vi "Teleop.vi"(10 "Match Info":T1={"Autonomous Elapsed Seconds"=0.0, "TeleOp Elapsed Seconds"=0.0, "Disabled Elapsed Seconds"=0.0, "Visited Autonomous"=FALSE, "Visited TeleOp"=FALSE, "Visited Disabled"=FALSE, "Autonomous Settings"={"Autonomous Style"=enum."Independent", "VI Refnum"=refnum}}, 11 "Call Context":T2) -> ()   [LabVIEW 2012]
doc: "This VI is called for each TeleOp packet received from the DS where the robot is not disabled. It is often used to read from the joysticks and update I/O or to update setpoints for timed control loops. It should complete and return within 20 milliseconds or it may miss DS packets."
uses:
  <vilib>/Rock Robotics/WPI/DriverStation/WPI_DriverStationDerivedRobotMode.ctl
  <vilib>/Rock Robotics/WPI/DriverStation/WPI_DriverStationMatch Info.ctl
  <vilib>/Rock Robotics/WPI/Relay/WPI_RelayValue.ctl
  Robot Global Data.vi
  <vilib>/Rock Robotics/WPI/Joystick/WPI_JoystickGetSetRefNum.vi
panel:
  in  "Ext Const":dbl=0.5
  in  "Dep Const":dbl=1.0
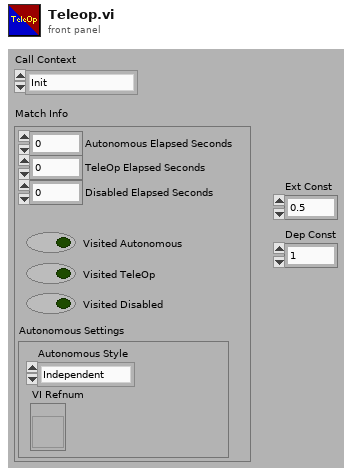
[diagram p1: front panel]
types:
  T1 = typedef "WPI_DriverStationMatch Info.ctl" = cluster{"Autonomous Elapsed Seconds":dbl, "TeleOp Elapsed Seconds":dbl, "Disabled Elapsed Seconds":dbl, "Visited Autonomous":bool, "Visited TeleOp":bool, "Visited Disabled":bool, "Autonomous Settings":cluster{"Autonomous Style":enum16{"Iterative", "Independent"}, "VI Refnum":refnum<vi>}}
  T2 = typedef "WPI_DriverStationDerivedRobotMode.ctl" = enum16{"Init", "Execute", "Stop"}
  T3 = typedef "WPI_RelayValue.ctl" = enum16{"Off", "On", "Forward", "Reverse"}
  T4 = cluster{"Driver Station Digital Input (1-8)[0]":bool, "Driver Station Digital Input (1-8)[1]":bool, "Driver Station Digital Input (1-8)[2]":bool, "Driver Station Digital Input (1-8)[3]":bool, "Driver Station Digital Input (1-8)[4]":bool, "Driver Station Digital Input (1-8)[5]":bool, "Driver Station Digital Input (1-8)[6]":bool, "Driver Station Digital Input (1-8)[7]":bool, "Driver Station Digital Input (1-8)[8]":bool}
  T5 = cluster{"Right Servo High":dbl, "Right Servo Mid":dbl, "Right Servo Low":dbl, "Left Servo High":dbl, "Left Servo Mid":dbl, "Left Servo Low":dbl}
  T6 = typedef "WPI_JoystickDevRef.ctl" = cluster{"Device":T7}
  T7 = typedef "WPI_JoystickDeviceEnum.ctl" = enum16{"USB 1", "USB 2", "USB 3", "USB 4", "Kinect 1", "Kinect 2"}
  T8 = cluster{"axis 1 (x)":dbl, "axis 2 (y)":dbl, "axis 3 (throttle)":dbl, "axis 4":dbl, "axis 5":dbl, "axis 6":dbl}
  T9 = typedef "WPI_ServoDeviceRef.ctl" = cluster{"DeviceStatus":errorcluster, "Digital Module":T10, "PWM Channel":T11, "DeadBand":T12}
  T10 = typedef "FPGA_TypedefDigitalModule.ctl" = enum16{"Digital Module 1", "Digital Module 2"}
  T11 = typedef "FPGA_DIOPWMChannel.ctl" = enum8{"PWM 1", "PWM 2", "PWM 3", "PWM 4", "PWM 5", "PWM 6", "PWM 7", "PWM 8", "PWM 9", "PWM 10", "Invalid"}
  T12 = typedef "WPI_PWMDeadband.ctl" = cluster{"Name":string, "maxPositivePwm":i32, "minPositivePwm":i32, "centerPwm":i32, "maxNegativePwm":i32, "minNegativePwm":i32, "angularRange":u16}
  T13 = typedef "WPI_MotorControlDeviceRef.ctl" = cluster{"DeviceStatus":errorcluster, "Type":enum16{"PWM", "CAN"}, "PWM":cluster{"Digital Module":T10, "PWM Channel":T11, "DeadBand":T12}, "CAN":cluster{"Device Number":u8, "Control Mode":T14, "Semaphore":T15, "Max Vout":dbl}, "Invert":bool, "TransformRef":T16, "InvTransformRef":T16}
  T14 = typedef "WPI_CANJaguar_ControlMode.ctl" = enum8{"Percent VBus", "Current", "Speed", "Position", "Voltage"}
  T15 = typedef "Semaphore RefNum" = refnum<k1>
  T16 = typedef "WPI_PWMTransform_ConPane.ctl" = refnum<vi>
  T17 = typedef "WPI_JoystickButtonState.ctl" = cluster{"Button 1":bool, "Button 2":bool, "Button 3":bool, "Button 4":bool, "Button 5":bool, "Button 6":bool, "Button 7":bool, "Button 8":bool, "Button 9":bool, "Button 10":bool, "Button 11":bool, "Button 12":bool}
  T18 = cluster{"FlipperLeftUp":dbl, "FlipperLeftDown":dbl, "FlipperRightUp":dbl, "FlipperRightDown":dbl, "KickerLeftBack":dbl, "KickerLeftForward":dbl, "KickerRightBack":dbl, "KickerRightForward":dbl}
  T19 = typedef "WPI_RelayDevRef.ctl" = cluster{"DevStatus":errorcluster, "Relay Channel":T20, "Digital Module":T10, "Relay Direction":T21}
  T20 = typedef "FPGA_DIORelayChannel.ctl" = enum8{"Relay 1", "Relay 2", "Relay 3", "Relay 4", "Relay 5", "Relay 6", "Relay 7", "Relay 8", "Invalid"}
  T21 = typedef "WPI_RelayDirection.ctl" = enum16{"Both directions", "Forward only", "Reverse only"}
  T22 = typedef "WPI_DigitalInputDevRef.ctl" = cluster{"DevStatus":errorcluster, "DIO Channel":T23, "Digital Module":T10}
  T23 = typedef "FPGA_DIOChannel.ctl" = enum8{"DIO 1", "DIO 2", "DIO 3", "DIO 4", "DIO 5", "DIO 6", "DIO 7", "DIO 8", "DIO 9", "DIO 10", "DIO 11", "DIO 12", "DIO 13", "DIO 14", "Invalid"}
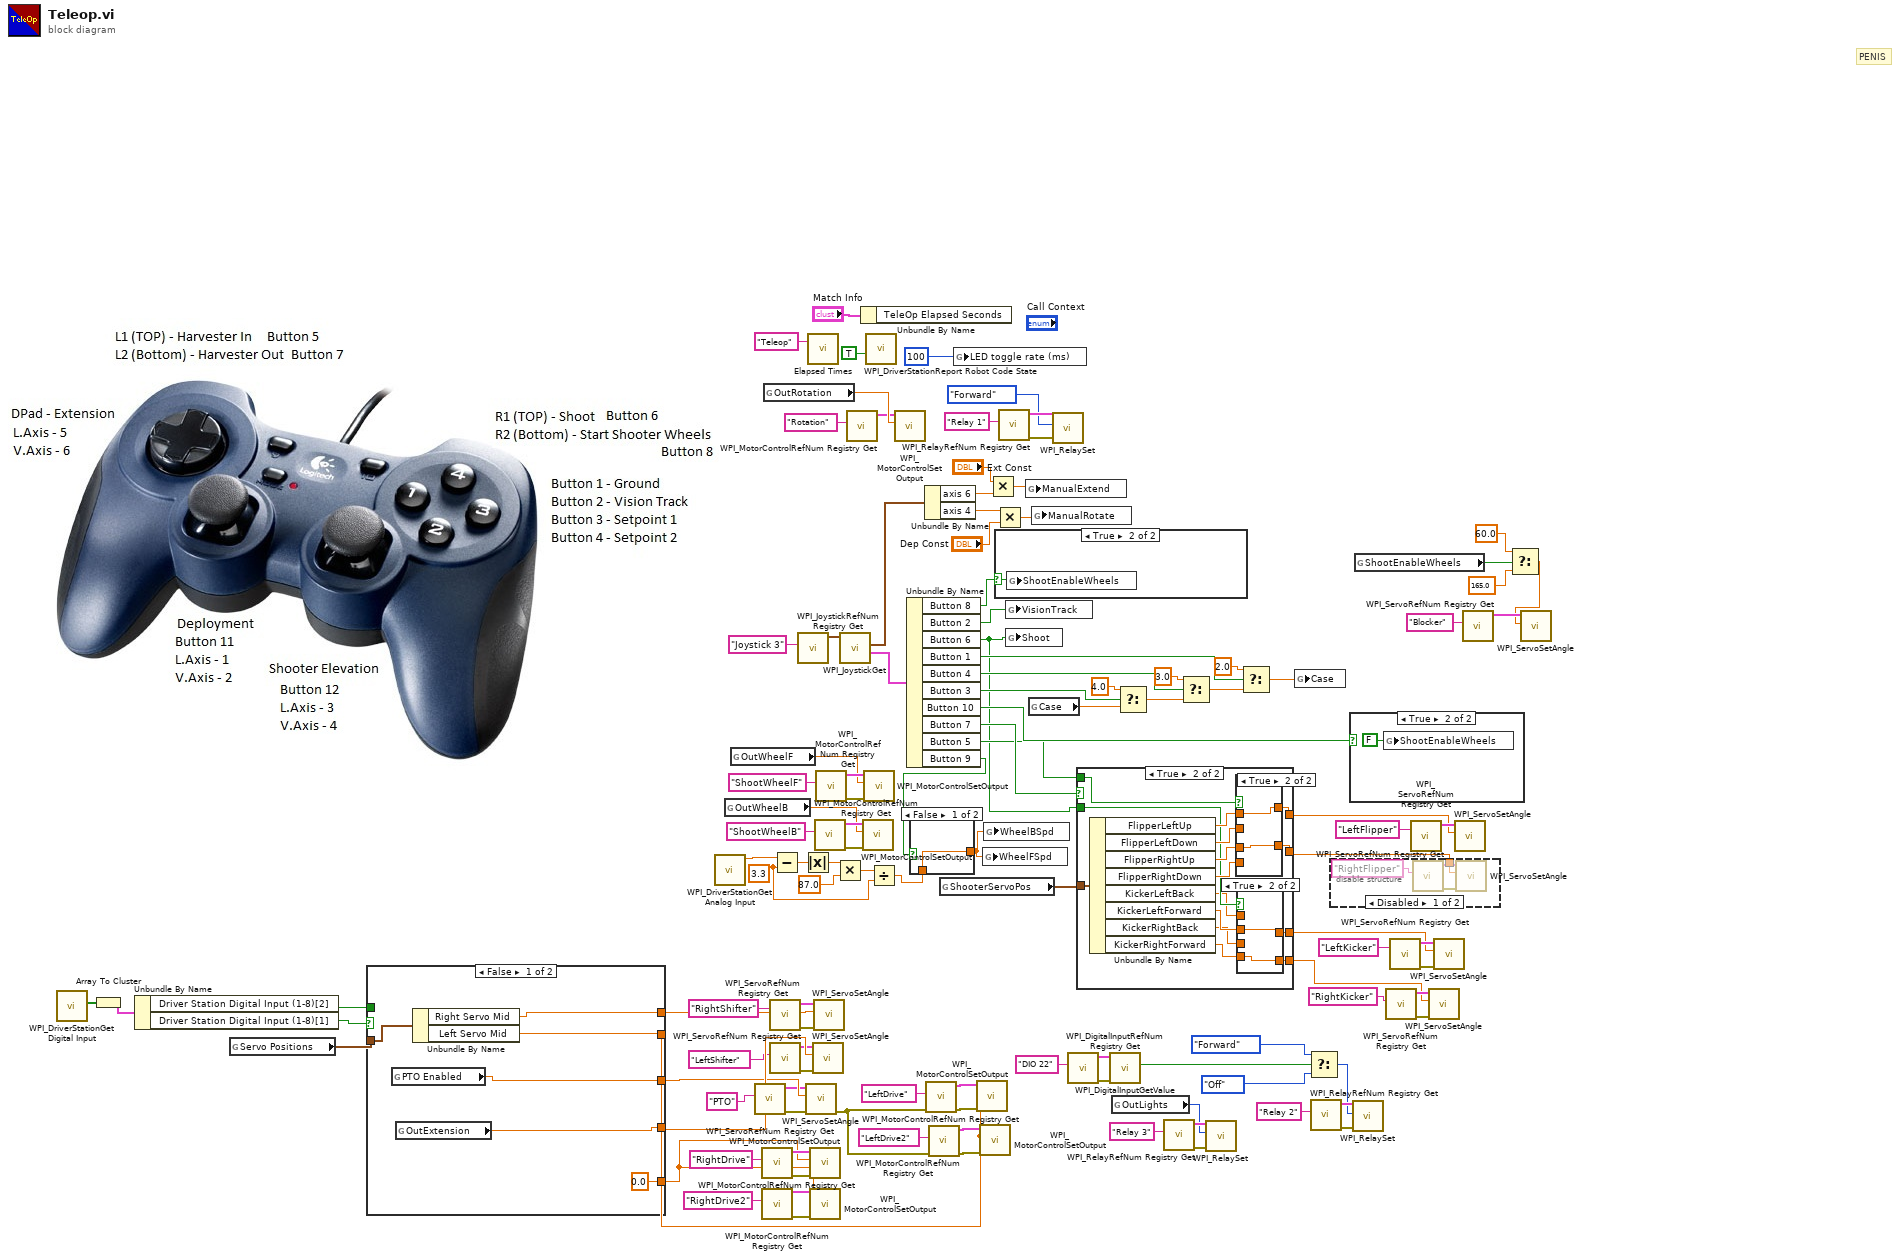
[diagram p0: block diagram]
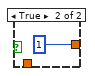
[diagram p2: hidden frame]
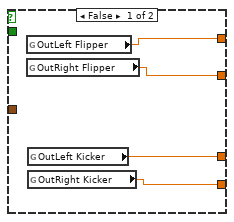
[diagram p4: hidden frame]
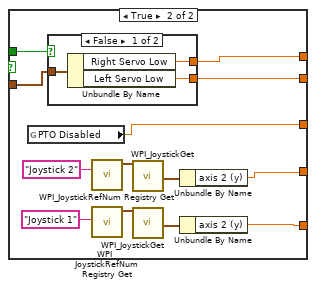
[diagram p7: hidden frame]
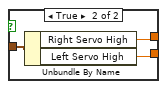
[diagram p8: hidden frame]
diagram:
  w2 = 3.3 ("y")
  # "PENIS"
  n1 = call <vilib>:"WPI_DriverStationGet Digital Input.vi"() -> ("Driver Station Digital Input (1-8)"=w87:bool[])  [unwired: 11 in]
  n2 = Array To Cluster(array=w87) -> (cluster=w86:T4)
  n3 = Unbundle By Name(w86) -> ("Driver Station Digital Input (1-8)[2]"=w85:bool, "Driver Station Digital Input (1-8)[1]"=w25:bool)
  n4 = global read "Robot Global Data.vi" "Servo Positions"() -> (w84:T5)
  n5 = case shown="False" w25 {
    tunnel: w85 -> [_ w138]
    tunnel: w84 -> [w125 w137]
    tunnel: [w124 w136] -> w83
    tunnel: [w123 w135] -> w82
    tunnel: [w122 w134] -> w75
    tunnel: [w120 w127] -> w74
    tunnel: [0.0 w126] -> w73
    frame False {
      n6 = global read "Robot Global Data.vi" "PTO Enabled"() -> (w122:dbl)
      n7 = global read "Robot Global Data.vi" "OutExtension"() -> (w120:dbl)
      n8 = Unbundle By Name(w125) -> ("Right Servo Mid"=w124:dbl, "Left Servo Mid"=w123:dbl)
    }
    frame True {
      n9 = global read "Robot Global Data.vi" "PTO Disabled"() -> (w134:dbl)
      n10 = case shown="False" w138 {
        tunnel: w137 -> [w141 w144]
        tunnel: [w140 w143] -> w136
        tunnel: [w139 w142] -> w135
        frame False {
          n11 = Unbundle By Name(w141) -> ("Right Servo Low"=w140:dbl, "Left Servo Low"=w139:dbl)
        }
        frame True {
          n12 = Unbundle By Name(w144) -> ("Right Servo High"=w143:dbl, "Left Servo High"=w142:dbl)
        }
      }
      n13 = call <vilib>:"WPI_JoystickRefNum Registry Get.vi"("refnum name"="Joystick 2") -> ("JoystickDevRef"=w128:T6)  [unwired: 1 in, 9 out]
      n14 = call <vilib>:"WPI_JoystickRefNum Registry Get.vi"("refnum name"="Joystick 1") -> ("JoystickDevRef"=w132:T6)  [unwired: 1 in, 9 out]
      n15 = call <vilib>:"WPI_JoystickGet.vi"("JoystickDevRef"=w128) -> ("Axes"=w130:T8)  [unwired: 1 in, 5 out]
      n16 = call <vilib>:"WPI_JoystickGet.vi"("JoystickDevRef"=w132) -> ("Axes"=w133:T8)  [unwired: 1 in, 5 out]
      n17 = Unbundle By Name(w130) -> ("axis 2 (y)"=w127:dbl)
      n18 = Unbundle By Name(w133) -> ("axis 2 (y)"=w126:dbl)
    }
  }
  n19 = call <vilib>:"WPI_DriverStationGet Analog Input.vi"() -> ("Analog 1 (V)"=w7:dbl)  [unwired: 8 in, 3 out]
  n20 = global read "Robot Global Data.vi" "OutWheelB"() -> (w45:dbl)
  n21 = global read "Robot Global Data.vi" "OutWheelF"() -> (w46:dbl)
  n22 = call <vilib>:"WPI_ServoRefNum Registry Get.vi"("refnum name"="PTO") -> ("error out"=w68:errorcluster, "ServoDeviceRef"=w69:T9)  [unwired: 9 in]
  n23 = call <vilib>:"WPI_MotorControlRefNum Registry Get.vi"("refnum name"="RightDrive") -> ("error out"=w97:errorcluster, "MotorControlDevRef"=w99:T13)  [unwired: 9 in]
  n24 = call <vilib>:"WPI_MotorControlRefNum Registry Get.vi"("refnum name"="RightDrive2") -> ("error out"=w90:errorcluster, "MotorControlDevRef"=w88:T13)  [unwired: 9 in]
  n25 = global read "Robot Global Data.vi" "OutRotation"() -> (w72:dbl)
  n26 = call <vilib>:"WPI_ServoRefNum Registry Get.vi"("refnum name"="RightShifter") -> ("error out"=w78:errorcluster, "ServoDeviceRef"=w79:T9)  [unwired: 9 in]
  n27 = call <vilib>:"WPI_ServoRefNum Registry Get.vi"("refnum name"="LeftShifter") -> ("error out"=w80:errorcluster, "ServoDeviceRef"=w81:T9)  [unwired: 9 in]
  n28 = Subtract(x=w7, y=w2) -> (x-y=w6:dbl)
  n29 = call <vilib>:"WPI_JoystickRefNum Registry Get.vi"("refnum name"="Joystick 3") -> ("JoystickDevRef"=w116:T6)  [unwired: 9 in, 1 out]
  n30 = Absolute Value(x=w6) -> (abs(x)=w5:dbl)
  n31 = call <vilib>:"WPI_ServoSetAngle.vi"("error in (no error)"=w68, "Angle"=w75, "ServoDeviceRef"=w69) -> ("error out"=w64:errorcluster)  [unwired: 7 in, 1 out]
  n32 = call "Elapsed Times.vi"("Call Name"="Teleop") -> ()  [unwired: 2 in, 1 out]
  n33 = call <vilib>:"WPI_MotorControlSetOutput.vi"("error in (no error)"=w97, "Output"=w73, "MotorControlDevRef"=w99) -> ()  [unwired: 6 in, 3 out]
  n34 = call <vilib>:"WPI_MotorControlSetOutput.vi"("error in (no error)"=w90, "Output"=w73, "MotorControlDevRef"=w88) -> ()  [unwired: 6 in, 3 out]
  n35 = call <vilib>:"WPI_ServoSetAngle.vi"("error in (no error)"=w80, "Angle"=w82, "ServoDeviceRef"=w81) -> ()  [unwired: 7 in, 2 out]
  n36 = call <vilib>:"WPI_ServoSetAngle.vi"("error in (no error)"=w78, "Angle"=w83, "ServoDeviceRef"=w79) -> ()  [unwired: 7 in, 2 out]
  n37 = call <vilib>:"WPI_MotorControlRefNum Registry Get.vi"("refnum name"="ShootWheelB") -> ("error out"=w48:errorcluster, "MotorControlDevRef"=w49:T13)  [unwired: 9 in]
  n38 = call <vilib>:"WPI_MotorControlRefNum Registry Get.vi"("refnum name"="ShootWheelF") -> ("error out"=w50:errorcluster, "MotorControlDevRef"=w47:T13)  [unwired: 9 in]
  n39 = Multiply(x=w5, y=87.0) -> (x*y=w3:dbl)
  n40 = call <vilib>:"WPI_JoystickGet.vi"("JoystickDevRef"=w116) -> ("Buttons"=w114:T17, "Axes"=w113:T8)  [unwired: 4 in, 1 out]
  n41 = call <vilib>:"WPI_MotorControlRefNum Registry Get.vi"("refnum name"="Rotation") -> ("MotorControlDevRef"=w70:T13)  [unwired: 9 in, 1 out]
  n42 = Unbundle By Name("Match Info") -> ()  [unwired: 1 out]
  n43 = call <vilib>:"WPI_MotorControlSetOutput.vi"("error in (no error)"=w48, "Output"=w45, "MotorControlDevRef"=w49) -> ()  [unwired: 6 in, 3 out]
  n44 = call <vilib>:"WPI_MotorControlSetOutput.vi"("error in (no error)"=w50, "Output"=w46, "MotorControlDevRef"=w47) -> ()  [unwired: 6 in, 3 out]
  n45 = call <vilib>:"WPI_DriverStationReport Robot Code State.vi"("TeleOp"=TRUE ("Autonomous")) -> ()  [unwired: 10 in, 1 out]
  n46 = Divide(x=w3, y=w2) -> (x/y=w1:dbl)
  n47 = call <vilib>:"WPI_MotorControlSetOutput.vi"("Output"=w72, "MotorControlDevRef"=w70) -> ()  [unwired: 7 in, 3 out]
  n48 = Unbundle By Name(w114) -> ("Button 8"=w101:bool, "Button 2"=w112:bool, "Button 6"=w29:bool, "Button 1"=w111:bool, "Button 4"=w109:bool, "Button 3"=w108:bool, "Button 10"=w44:bool, "Button 7"=w43:bool, "Button 5"=w42:bool, "Button 9"=w26:bool)
  n49 = case shown="False" w26 {
    tunnel: [w145 1] -> w27
    tunnel: w1 -> [w145 _]
    frame False {
    }
    frame True {
    }
  }
  n50 = Unbundle By Name(w113) -> ("axis 6"=w55:dbl, "axis 4"=w65:dbl)
  n51 = call <vilib>:"WPI_MotorControlRefNum Registry Get.vi"("error in (no error)"=w64, "refnum name"="LeftDrive") -> ("error out"=w92:errorcluster, "MotorControlDevRef"=w95:T13)  [unwired: 8 in]
  n52 = call <vilib>:"WPI_MotorControlRefNum Registry Get.vi"("error in (no error)"=w64, "refnum name"="LeftDrive2") -> ("error out"=w91:errorcluster, "MotorControlDevRef"=w93:T13)  [unwired: 8 in]
  n53 = global read "Robot Global Data.vi" "ShooterServoPos"() -> (w30:T18)
  n54 = global write "Robot Global Data.vi" "LED toggle rate (ms)"(u32 100 ("LED ms toggle rate")) -> ()
  n55 = call <vilib>:"WPI_MotorControlSetOutput.vi"("error in (no error)"=w92, "Output"=w74, "MotorControlDevRef"=w95) -> ()  [unwired: 6 in, 3 out]
  n56 = call <vilib>:"WPI_MotorControlSetOutput.vi"("error in (no error)"=w91, "Output"=w74, "MotorControlDevRef"=w93) -> ()  [unwired: 6 in, 3 out]
  n57 = global write "Robot Global Data.vi" "WheelFSpd"(w27) -> ()
  n58 = global write "Robot Global Data.vi" "WheelBSpd"(w27) -> ()
  n59 = Multiply(x="Ext Const", y=w55) -> (x*y=w53:dbl)
  n60 = Multiply(x=w65, y="Dep Const") -> (x*y=w63:dbl)
  n61 = case shown="True" w101 {
    selector: w101 -> [_ w147]
    frame False {
    }
    frame True {
      n62 = global write "Robot Global Data.vi" "ShootEnableWheels"(w147) -> ()
    }
  }
  n63 = call <vilib>:"WPI_RelayRefNum Registry Get.vi"("refnum name"="Relay 1") -> ("error out"=w60:errorcluster, "RelayDevRef"=w62:T19)  [unwired: 9 in]
  n64 = global write "Robot Global Data.vi" "VisionTrack"(w112) -> ()
  n65 = global write "Robot Global Data.vi" "Shoot"(w29) -> ()
  n66 = global write "Robot Global Data.vi" "ManualExtend"(w53) -> ()
  n67 = global read "Robot Global Data.vi" "Case"() -> (w103:dbl)
  n68 = global write "Robot Global Data.vi" "ManualRotate"(w63) -> ()
  n69 = call <vilib>:"WPI_RelaySet.vi"("error in (no error)"=w60, "RelayValue"=WPI_RelayValue."Forward", "RelayDevRef"=w62) -> ()  [unwired: 7 in, 2 out]
  n70 = call <vilib>:"WPI_DigitalInputRefNum Registry Get.vi"("refnum name"="DIO 22") -> ("error out"=w19:errorcluster, "DigitalInputDevRef"=w15:T22)  [unwired: 9 in]
  n71 = case shown="True" w43 {
    tunnel: w42 -> [_ w152]
    tunnel: [w151 w165] -> w33
    tunnel: [w150 w163] -> w32
    tunnel: [w149 w154] -> w31
    tunnel: [w148 w153] -> w28
    tunnel: w30 -> [_ w166]
    tunnel: w29 -> [_ w159]
    frame False {
      n72 = global read "Robot Global Data.vi" "OutLeft Flipper"() -> (w151:dbl)
      n73 = global read "Robot Global Data.vi" "OutRight Flipper"() -> (w150:dbl)
      n74 = global read "Robot Global Data.vi" "OutLeft Kicker"() -> (w149:dbl)
      n75 = global read "Robot Global Data.vi" "OutRight Kicker"() -> (w148:dbl)
    }
    frame True {
      n76 = Unbundle By Name(w166) -> ("FlipperLeftUp"=w164:dbl, "FlipperLeftDown"=w161:dbl, "FlipperRightUp"=w162:dbl, "FlipperRightDown"=w160:dbl, "KickerLeftBack"=w158:dbl, "KickerLeftForward"=w157:dbl, "KickerRightBack"=w156:dbl, "KickerRightForward"=w155:dbl)
      n77 = case shown="True" w152 {
        tunnel: [w172 w174] -> w165
        tunnel: w164 -> [_ w174]
        tunnel: [w171 w173] -> w163
        tunnel: w162 -> [_ w173]
        tunnel: w161 -> [w172 _]
        tunnel: w160 -> [w171 _]
        frame False {
        }
        frame True {
        }
      }
      n78 = case shown="True" w159 {
        tunnel: w158 -> [w168 _]
        tunnel: w157 -> [_ w169]
        tunnel: w156 -> [w167 _]
        tunnel: w155 -> [_ w170]
        tunnel: [w168 w169] -> w154
        tunnel: [w167 w170] -> w153
        frame False {
        }
        frame True {
        }
      }
    }
  }
  n79 = call <vilib>:"WPI_DigitalInputGetValue.vi"("error in (no error)"=w19, "DigitalInputDevRef"=w15) -> ("Value"=w18:bool)  [unwired: 7 in, 2 out]
  n80 = global read "Robot Global Data.vi" "OutLights"() -> (w24:T3)
  n81 = Select(t=4.0, s=w108, f=w103) -> (s? t:f=w107:dbl)
  n82 = call <vilib>:"WPI_RelayRefNum Registry Get.vi"("refnum name"="Relay 3") -> ("error out"=w58:errorcluster, "RelayDevRef"=w56:T19)  [unwired: 9 in]
  n83 = Select(t=3.0, s=w109, f=w107) -> (s? t:f=w105:dbl)
  n84 = call <vilib>:"WPI_RelaySet.vi"("error in (no error)"=w58, "RelayValue"=w24, "RelayDevRef"=w56) -> ()  [unwired: 7 in, 2 out]
  n85 = Select(t=2.0, s=w111, f=w105) -> (s? t:f=w102:dbl)
  n86 = global write "Robot Global Data.vi" "Case"(w102) -> ()
  n87 = Select(t=WPI_RelayValue."Forward" ("RelayValue"), s=w18, f=WPI_RelayValue."Off" ("RelayValue")) -> (s? t:f=w14:T3)
  n88 = call <vilib>:"WPI_RelayRefNum Registry Get.vi"("refnum name"="Relay 2") -> ("error out"=w21:errorcluster, "RelayDevRef"=w23:T19)  [unwired: 9 in]
  n89 = disable-structure shown="Disabled" {
    disable-tunnel: w32 -> [w175 _]
    frame Disabled {
      n90 = call <vilib>:"WPI_ServoRefNum Registry Get.vi"("refnum name"="RightFlipper") -> ("error out"=w178:errorcluster, "ServoDeviceRef"=w176:T9)  [unwired: 9 in]
      n91 = call <vilib>:"WPI_ServoSetAngle.vi"("error in (no error)"=w178, "Angle"=w175, "ServoDeviceRef"=w176) -> ()  [unwired: 7 in, 2 out]
    }
    frame Enabled {
    }
  }
  n92 = case shown="True" w44 {
    frame False {
    }
    frame True {
      n93 = global write "Robot Global Data.vi" "ShootEnableWheels"(FALSE ("ShootStartWheels")) -> ()
    }
  }
  n94 = call <vilib>:"WPI_RelaySet.vi"("error in (no error)"=w21, "RelayValue"=w14, "RelayDevRef"=w23) -> ()  [unwired: 7 in, 2 out]
  n95 = global read "Robot Global Data.vi" "ShootEnableWheels"() -> (w11:bool)
  n96 = call <vilib>:"WPI_ServoRefNum Registry Get.vi"("refnum name"="RightKicker") -> ("error out"=w40:errorcluster, "ServoDeviceRef"=w38:T9)  [unwired: 9 in]
  n97 = call <vilib>:"WPI_ServoRefNum Registry Get.vi"("refnum name"="LeftKicker") -> ("error out"=w34:errorcluster, "ServoDeviceRef"=w35:T9)  [unwired: 9 in]
  n98 = call <vilib>:"WPI_ServoRefNum Registry Get.vi"("refnum name"="LeftFlipper") -> ("ServoDeviceRef"=w36:T9)  [unwired: 9 in, 1 out]
  n99 = call <vilib>:"WPI_ServoSetAngle.vi"("error in (no error)"=w40, "Angle"=w28, "ServoDeviceRef"=w38) -> ()  [unwired: 7 in, 2 out]
  n100 = call <vilib>:"WPI_ServoSetAngle.vi"("error in (no error)"=w34, "Angle"=w31, "ServoDeviceRef"=w35) -> ()  [unwired: 7 in, 2 out]
  n101 = call <vilib>:"WPI_ServoSetAngle.vi"("Angle"=w33, "ServoDeviceRef"=w36) -> ()  [unwired: 8 in, 2 out]
  n102 = call <vilib>:"WPI_ServoRefNum Registry Get.vi"("refnum name"="Blocker") -> ("ServoDeviceRef"=w12:T9)  [unwired: 9 in, 1 out]
  n103 = Select(t=60.0 ("f"), s=w11, f=165.0 ("t")) -> (s? t:f=w10:dbl)
  n104 = call <vilib>:"WPI_ServoSetAngle.vi"("Angle"=w10, "ServoDeviceRef"=w12) -> ()  [unwired: 8 in, 2 out]
